vi "Script Flat to Rich Oneof Conversion.vi"(5 "message element metadata":T1={"Field Name"="", "Embedded Message Name"="", "Protobuf Index"=1, "MessageElementType"=enum."StringValue", "Repeated"=FALSE, "Is in Oneof"=FALSE, "Oneof Container Name"=""}, 7 "library in":refnum<vi>, 8 "error in (no error)":errorcluster, 9 "unbundler":refnum<vi>, 10 "bundler":refnum<vi>, 11 "vi in":refnum<vi>) -> (0 "error out":errorcluster, 3 "vi out":refnum<vi>)   [LabVIEW 2019, in "gRPC Template Creation Utility.lvlib"]
uses:
  gRPC Template Creation Utility.lvlib
  OneOf Constants/OneOfConstantsEnum.ctl
  TypeDefs/Message Element Type.ctl
  TypeDefs/Message Element Metadata (Scripting).ctl
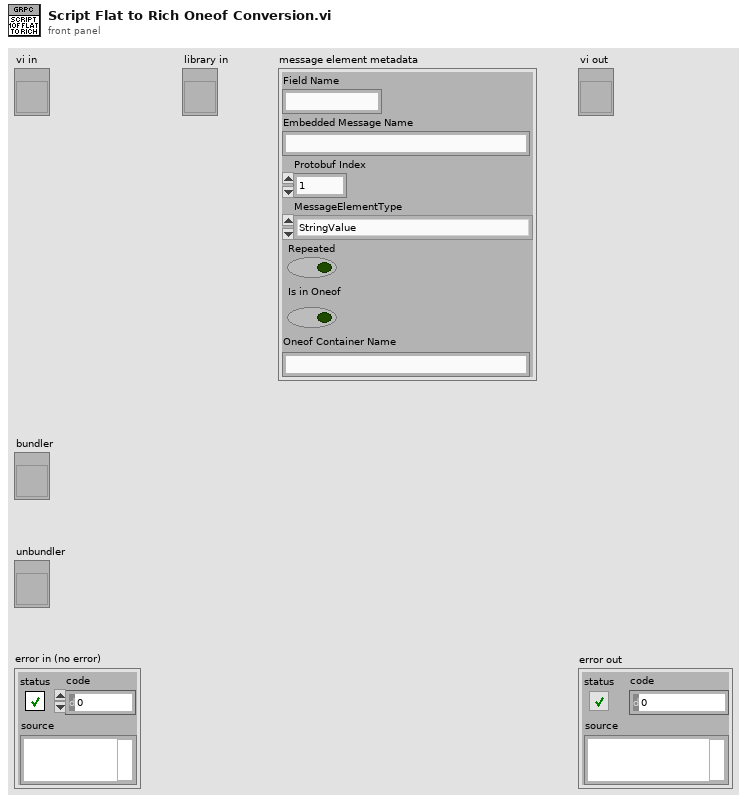
[diagram p1: front panel]
types:
  T1 = typedef "gRPC Template Creation Utility.lvlib/Message Element Metadata (Scripting).ctl" = cluster{"Field Name":string, "Embedded Message Name":string, "Protobuf Index":i32, "MessageElementType":T2, "Repeated":bool, "Is in Oneof":bool, "Oneof Container Name":string}
  T2 = typedef "gRPC Template Creation Utility.lvlib/Message Element Type.ctl" = enum32{"Int32Value", "FloatValue", "DoubleValue", "BoolValue", "StringValue", "MessageValue", "Int64Value", "UInt32Value", "UInt64Value", "EnumValue", "Bytes", "Fixed64", "Fixed32", "SFixed64", "SFixed32", "SInt64", "SInt32"}
  T3 = typedef "gRPC Template Creation Utility.lvlib/OneOfConstantsEnum.ctl" = enum16{"FlatToRichVIPrefix", "RichToFlatVIPrefix", "FlatTypeDefSuffix"}
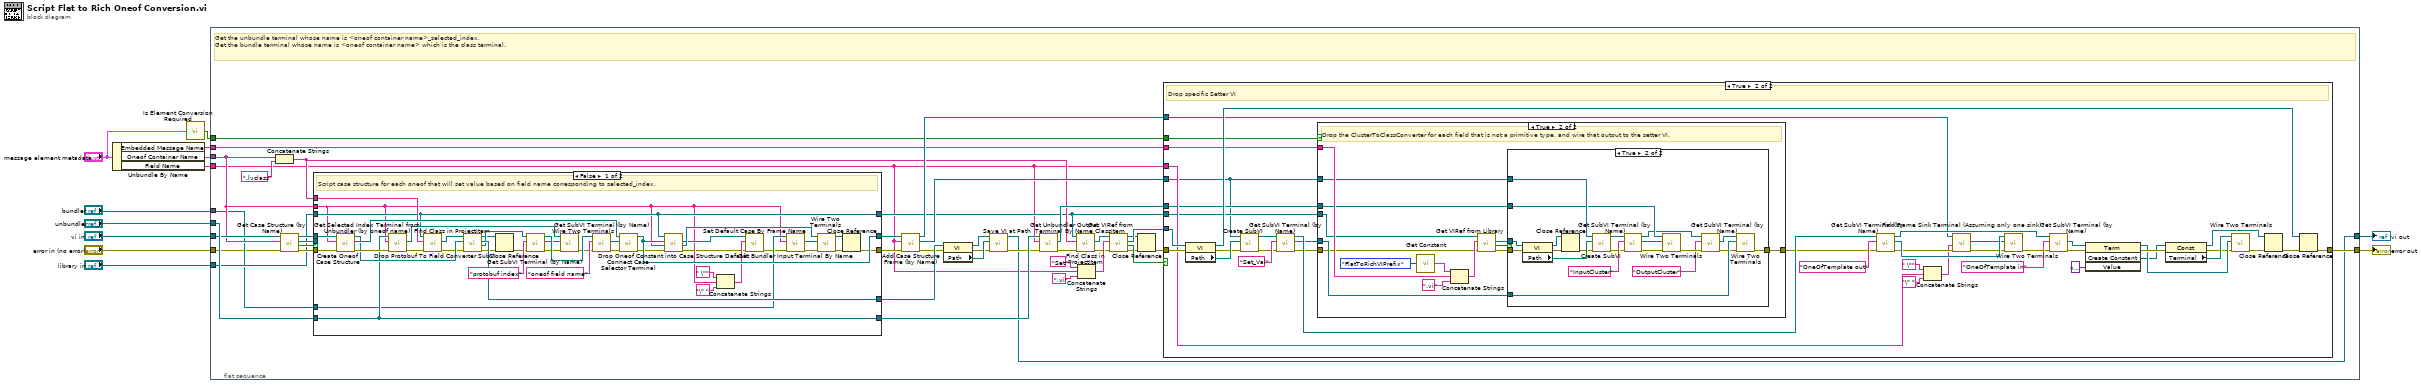
[diagram p0: block diagram]
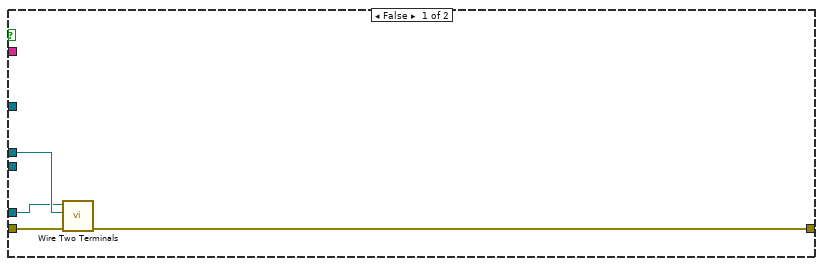
[diagram p3: hidden frame]
diagram:
  n1 = Unbundle By Name("message element metadata") -> ("Embedded Message Name"=w10:string, "Oneof Container Name"=w12:string, "Field Name"=w11:string)
  n2 = call "Is Element Conversion Required.vi"("element metadata"="message element metadata") -> ("conversion required"=w1:bool)
  n3 = flat-sequence {
    tunnel: w12 -> [w40]
    tunnel: w11 -> [w16]
    tunnel: "error in (no error)" -> [w17]
    tunnel: [w39] -> w4
    tunnel: "bundler" -> [w18]
    tunnel: "unbundler" -> [w53]
    tunnel: "vi in" -> [w52]
    tunnel: "library in" -> [w38]
    tunnel: [w32] -> w3
    tunnel: w1 -> [w26]
    tunnel: w10 -> [w25]
    frame #0 {
      # "Get the unbundle terminal whose name is <oneof container name>_selected_index.\nGet the bundle terminal whose name is <oneof container name> which is the class terminal."
      n4 = Concatenate Strings(w40, ".lvclass" ("string")) -> (w28:string)
      n5 = call "Get Case Structure (by Name).vi"("error in (no error)"=w17, "Case Structure name"=w40, "VI ref in"=w52) -> ("error out"=w46:errorcluster, "Found ?"=w50:bool, "CaseStructure out"=w47:refnum<vi>, "VI ref out"=w51:refnum<vi>)  [unwired: 5 in]
      n6 = case shown="False" w50 {
        tunnel: w53 -> [w147 w180]
        tunnel: w40 -> [w145 _]
        tunnel: w51 -> [w176 w178]
        tunnel: [w160 w181] -> w45
        tunnel: w47 -> [_ w181]
        tunnel: [w147 w180] -> w42
        tunnel: [w141 w179] -> w43
        tunnel: w46 -> [w143 w179]
        tunnel: [w172 w178] -> w36
        tunnel: w38 -> [w148 w177]
        tunnel: [w148 w177] -> w24
        tunnel: w28 -> [w149 _]
        tunnel: w18 -> [w146 _]
        frame False {
          # "Script case structure for each oneof that will set value based on field name corresponding to selected_index."
          n7 = call "Create Oneof Case Structure.vi"("error in (no error)"=w143, "Oneof Container Name"=w145, "VI in"=w176) -> ("error out"=w174:errorcluster, "CaseStructure out"=w175:refnum<vi>, "VI out"=w173:refnum<vi>)  [unwired: 6 in]
          n8 = call "Get Selected Index Terminal from Unbundler (by oneof name).vi"("error in (no error)"=w174, "Oneof Container Name"=w145, "Unbundler in"=w147) -> ("error out"=w151:errorcluster, "Terminal Refnum"=w166:refnum<vi>)  [unwired: 5 in, 2 out]
          n9 = call "Find Class in ProjectItem.vi"("error in (no error)"=w151, "Class Name"=w149, "ProjectItem in"=w148) -> ("error out"=w150:errorcluster, "LVClass out"=w152:refnum<vi>)  [unwired: 5 in, 2 out]
          n10 = call "Drop Protobuf To Field Converter SubVI.vi"("error in (no error)"=w150, "Owner VI in"=w173, "Library"=w152) -> ("error out"=w138:errorcluster, "SubVI out"=w171:refnum<vi>, "Owner VI out"=w172:refnum<vi>, "Library out"=w137:refnum<vi>)  [unwired: 5 in]
          n11 = Close Reference(reference=w137, error in (no error)=w138) -> (error out=w136:errorcluster)
          n12 = call "Get SubVI Terminal (by Name).vi"("error in (no error)"=w136, "Terminal name"="protobuf index", "SubVI in"=w171) -> ("error out"=w163:errorcluster, "SubVI Term ref"=w165:refnum<vi>, "SubVI out"=w168:refnum<vi>)  [unwired: 5 in, 1 out]
          n13 = call "Wire Two Terminals.vi"("error in (no error)"=w163, "Sink Terminal in"=w165, "Source Terminal"=w166) -> ("error out"=w162:errorcluster)  [unwired: 7 in, 1 out]
          n14 = call "Get SubVI Terminal (by Name).vi"("error in (no error)"=w162, "Terminal name"="oneof field name", "SubVI in"=w168) -> ("error out"=w167:errorcluster, "SubVI Term ref"=w164:refnum<vi>)  [unwired: 5 in, 2 out]
          n15 = call "Connect Case Selector Terminal.vi"("error in (no error)"=w167, "Wire Source"=w164, "Case Structure in"=w175) -> ("error IO"=w159:errorcluster, "Case Structure out"=w160:refnum<vi>)  [unwired: 7 in]
          n16 = call "Drop Oneof Constant into Case Structure Default.vi"("error in (no error)"=w159, "Oneof Container Name"=w145, "CaseStructure in"=w160, "Library in"=w148) -> ("error out"=w140:errorcluster, "LVClass Constant Terminal out"=w161:refnum<vi>, "CaseStructure out"=w153:refnum<vi>)  [unwired: 4 in, 1 out]
          n17 = Concatenate Strings(" \"" ("string"), w145, "\" " ("string")) -> (w156:string)
          n18 = call "Set Default Case By Frame Name.vi"("error in (no error)"=w140, "Frame Name"=w156, "CaseStructure in"=w153) -> ("error out"=w139:errorcluster)  [unwired: 7 in, 1 out]
          n19 = call "Get Bundler Input Terminal By Name.vi"("error in (no error)"=w139, "Terminal name"=w145, "Bundler in"=w146) -> ("error out"=w142:errorcluster, "Terminal Refnum"=w144:refnum<vi>)  [unwired: 5 in, 2 out]
          n20 = call "Wire Two Terminals.vi"("error in (no error)"=w142, "Sink Terminal in"=w144, "Source Terminal"=w161) -> ("error out"=w158:errorcluster, "Source Terminal out"=w157:refnum<vi>)  [unwired: 7 in]
          n21 = Close Reference(reference=w157, error in (no error)=w158) -> (error out=w141:errorcluster)
        }
        frame True {
        }
      }
      n22 = call "Add Case Structure Frame (by Name).vi"("error in (no error)"=w43, "Frame name"=w16, "CaseStructure in"=w45) -> ("error out"=w31:errorcluster, "Case Frame"=w44:refnum<vi>, "CaseStructure out"=w37:refnum<vi>)  [unwired: 6 in]
      n23 = property class="VI"(reference=w36, error in=w31) -> (reference out=w34:refnum<vi>, error out=w30:errorcluster, "Path"=w33:path)
      n24 = call "Save VI at Path.vi"("error in (no error)"=w30, "Path"=w33, "VI in"=w34) -> ("error out"=w35:errorcluster, "VI out"=w32:refnum<vi>)  [unwired: 6 in, 1 out]
      n25 = call "Get Unbundler Output Terminal By Name.vi"("error in (no error)"=w35, "Terminal name"=w16, "Unbundler in"=w42) -> ("error out"=w27:errorcluster, "Terminal Refnum"=w41:refnum<vi>)  [unwired: 5 in, 2 out]
      n26 = call "Find Class in ProjectItem.vi"("error in (no error)"=w27, "Class Name"=w28, "ProjectItem in"=w24) -> ("error out"=w21:errorcluster, "LVClass out"=w23:refnum<vi>)  [unwired: 5 in, 2 out]
      n27 = Concatenate Strings("Set" ("string"), w16, ".vi" ("string")) -> (w22:string)
      n28 = call "Get VIRef from ClassItem.vi"("error in (no error)"=w21, "item name"=w22, "class in"=w23) -> ("error out"=w15:errorcluster, "found"=w19:bool, "vi"=w20:refnum<vi>, "class out"=w14:refnum<vi>)  [unwired: 5 in]
      n29 = Close Reference(reference=w14, error in (no error)=w15) -> (error out=w13:errorcluster)
      n30 = case shown="True" w19 {
        tunnel: w20 -> [_ w96]
        tunnel: w44 -> [_ w55]
        tunnel: w41 -> [_ w58]
        tunnel: w13 -> [w54 w79]
        tunnel: [w54 w75] -> w39
        tunnel: w16 -> [_ w72]
        tunnel: w37 -> [_ w71]
        tunnel: w26 -> [_ w63]
        tunnel: w25 -> [_ w62]
        tunnel: w24 -> [_ w60]
        frame False {
        }
        frame True {
          # "Drop specific Setter VI"
          n31 = property class="VI"(reference=w96, error in=w79) -> (reference out=w76:refnum<vi>, error out=w80:errorcluster, "Path"=w95:path)
          n32 = call "Create SubVI.vi"("error in (no error)"=w80, "Path"=w95, "Diagram in"=w55) -> ("error out"=w82:errorcluster, "subVI refnum"=w94:refnum<vi>)  [unwired: 7 in]
          n33 = call "Get SubVI Terminal (by Name).vi"("error in (no error)"=w82, "Terminal name"="Set_Val", "SubVI in"=w94) -> ("error out"=w59:errorcluster, "SubVI Term ref"=w57:refnum<vi>, "SubVI out"=w92:refnum<vi>)  [unwired: 5 in, 1 out]
          n34 = case shown="True" w63 {
            tunnel: w62 -> [_ w112]
            tunnel: w60 -> [_ w111]
            tunnel: w59 -> [w100 w103]
            tunnel: w58 -> [w99 w106]
            tunnel: w57 -> [w98 w105]
            tunnel: [w97 w104] -> w56
            tunnel: w55 -> [_ w107]
            frame False {
              n35 = call "Wire Two Terminals.vi"("error in (no error)"=w100, "Sink Terminal in"=w99, "Source Terminal"=w98) -> ("error out"=w97:errorcluster)  [unwired: 7 in, 1 out]
            }
            frame True {
              # "Drop the ClusterToClassConverter for each field that is not a primitive type, and wire that output to the setter VI."
              n36 = call "Get Constant.vi"("Selection"=OneOfConstantsEnum."FlatToRichVIPrefix") -> ("String"=w101:string)
              n37 = Concatenate Strings(w101, w112, ".vi" ("string")) -> (w113:string)
              n38 = call "Get VIRef from Library.vi"("error in (no error)"=w103, "item name"=w113, "library in"=w111) -> ("error out"=w108:errorcluster, "found"=w110:bool, "vi"=w109:refnum<vi>)  [unwired: 5 in, 1 out]
              n39 = case shown="True" w110 {
                tunnel: w109 -> [_ w135]
                tunnel: w108 -> [w115 w134]
                tunnel: w107 -> [_ w132]
                tunnel: w106 -> [_ w128]
                tunnel: w105 -> [_ w122]
                tunnel: [w115 w119] -> w104
                frame False {
                }
                frame True {
                  n40 = property class="VI"(reference=w135, error in=w134) -> (reference out=w117:refnum<vi>, error out=w118:errorcluster, "Path"=w133:path)
                  n41 = Close Reference(reference=w117, error in (no error)=w118) -> (error out=w116:errorcluster)
                  n42 = call "Create SubVI.vi"("error in (no error)"=w116, "Path"=w133, "Diagram in"=w132) -> ("error out"=w129:errorcluster, "subVI refnum"=w130:refnum<vi>)  [unwired: 7 in]
                  n43 = call "Get SubVI Terminal (by Name).vi"("error in (no error)"=w129, "Terminal name"="InputCluster", "SubVI in"=w130) -> ("error out"=w126:errorcluster, "SubVI Term ref"=w127:refnum<vi>, "SubVI out"=w124:refnum<vi>)  [unwired: 5 in, 1 out]
                  n44 = call "Wire Two Terminals.vi"("error in (no error)"=w126, "Sink Terminal in"=w127, "Source Terminal"=w128) -> ("error out"=w125:errorcluster)  [unwired: 7 in, 1 out]
                  n45 = call "Get SubVI Terminal (by Name).vi"("error in (no error)"=w125, "Terminal name"="OutputCluster", "SubVI in"=w124) -> ("error out"=w120:errorcluster, "SubVI Term ref"=w121:refnum<vi>)  [unwired: 5 in, 2 out]
                  n46 = call "Wire Two Terminals.vi"("error in (no error)"=w120, "Sink Terminal in"=w122, "Source Terminal"=w121) -> ("error out"=w119:errorcluster)  [unwired: 7 in, 1 out]
                }
              }
            }
          }
          n47 = call "Get SubVI Terminal (by Name).vi"("error in (no error)"=w56, "Terminal name"="OneOfTemplate out", "SubVI in"=w92) -> ("error out"=w68:errorcluster, "SubVI Term ref"=w70:refnum<vi>, "SubVI out"=w81:refnum<vi>)  [unwired: 5 in, 1 out]
          n48 = Concatenate Strings(" \"" ("string"), w72, "\" " ("string")) -> (w66:string)
          n49 = call "Find Frame Sink Terminal (Assuming only one sink).vi"("error in (no error)"=w68, "Frame Name"=w66, "CaseStructure in"=w71) -> ("error IO"=w67:errorcluster, "Terminal ref"=w69:refnum<vi>)  [unwired: 5 in, 2 out]
          n50 = call "Wire Two Terminals.vi"("error in (no error)"=w67, "Sink Terminal in"=w69, "Source Terminal"=w70) -> ("error out"=w87:errorcluster)  [unwired: 7 in, 1 out]
          n51 = call "Get SubVI Terminal (by Name).vi"("error in (no error)"=w87, "Terminal name"="OneOfTemplate in", "SubVI in"=w81) -> ("error out"=w86:errorcluster, "SubVI Term ref"=w89:refnum<vi>)  [unwired: 5 in, 2 out]
          n52 = invoke class="Term" method="Create Constant"(reference=w89, error in=w86, "Value"=variant) -> (reference out=w83:refnum<vi>, error out=w85:errorcluster, "Create Constant"=w61:refnum<vi>)  [unwired: 1 in, 1 out]
          n53 = property class="Const"(reference=w61, error in=w85) -> (reference out=w78:refnum<vi>, error out=w74:errorcluster, "Terminal"=w84:refnum<vi>)
          n54 = call "Wire Two Terminals.vi"("error in (no error)"=w74, "Sink Terminal in"=w83, "Source Terminal"=w84) -> ("error out"=w73:errorcluster)  [unwired: 7 in, 1 out]
          n55 = Close Reference(reference=w78, error in (no error)=w73) -> (error out=w77:errorcluster)
          n56 = Close Reference(reference=w76, error in (no error)=w77) -> (error out=w75:errorcluster)
        }
      }
    }
  }
  "error out" <- w4
  "vi out" <- w3
